vi "CheckGameBoardQueueLogic.vi"(8 "error in (no error)":errorcluster, 9 "Current Color in":i32, 10 "Coloring Board in":cluster{"tile":T1, "color":i8}[][](array[cluster]), 11 "Queue in":refnum<queue>) -> (0 "error out":errorcluster, 1 "Current Color out":i32, 2 "Coloring Board out":cluster{"tile":T1, "color":i8}[][](array[cluster]), 3 "Queue out":refnum<queue>)   [LabVIEW 2020]
uses:
  TypeDef/tiles-key-trunct.ctl
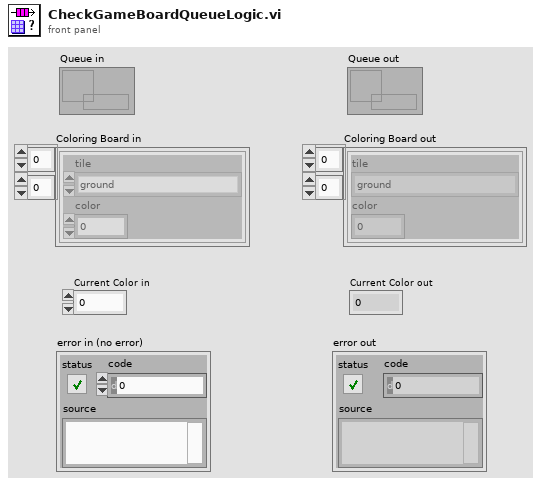
[diagram p1: front panel]
types:
  T1 = typedef "tiles-key-trunct.ctl" = enum16{"ground", "wall", "head (right)", "head (up)", "head (left)", "head (down)", "L-turn (right-up)", "L-turn (up-left)", "L-turn (left-down)", "L-turn (down-right)", "body (right)", "body (up)", "body (left)", "body (down)", "R-turn (right-down)", "R-turn (up-right)", "R-turn (left-up)", "R-turn (down-left)", "tail (right)", "tail (up)", "tail (left)", "tail (down)"}
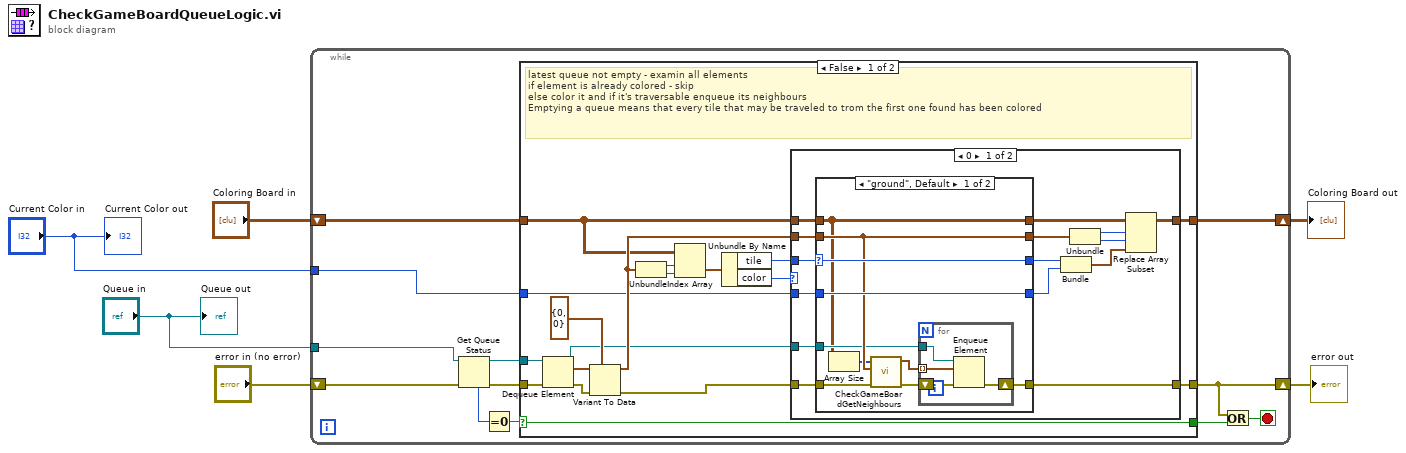
[diagram p0: block diagram]
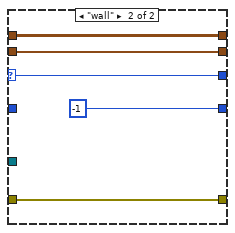
[diagram p2: hidden frame]
diagram:
  n1 = while {
    shift-right: [w11] -> w4
    shift-left: "error in (no error)" -> [w18]
    shift-right: [w14] -> w6
    shift-left: "Coloring Board in" -> [w13]
    tunnel: "Queue in" -> [w8]
    tunnel: "Current Color in" -> [w9]
    stop <- w10 stop-if-true
    n2 = Get Queue Status(queue=w8, error in (no error)=w18) -> (queue out=w7:refnum<queue>, error out=w15:errorcluster, # elements in queue=w17:i32)  [unwired: 1 in, 5 out]
    n3 = Equal To 0?(x=w17) -> (x = 0?=w16:bool)
    n4 = case shown="False" w16 {
      selector: w16 -> [w36 w73]
      tunnel: [w25 w75] -> w11
      tunnel: w15 -> [w34 w75]
      tunnel: [w19 w74] -> w14
      tunnel: w13 -> [w22 w74]
      tunnel: [w36 w73] -> w12
      tunnel: w7 -> [w35 _]
      tunnel: w9 -> [w20 _]
      frame False {
        # "latest queue not empty - examin all elements\nif element is already colored - skip \nelse color it and if it's traversable enqueue its neighbours\nEmptying a queue means that every tile that may be traveled to trom the first one found has been colored"
        n5 = Dequeue Element(queue=w35, error in (no error)=w34) -> (queue out=w21:refnum<queue>, element=w32:cluster{"row":i32, "col":i32}, error out=w33:errorcluster)  [unwired: 1 in, 1 out]
        n6 = Variant To Data(error in=w33, type=cluster{"row":i32, "col":i32} {"row"=0, "col"=0} ("cluster"), Variant=w32) -> (data=w23:cluster{"row":i32, "col":i32}, error out=w26:errorcluster)
        n7 = Unbundle(w23) -> ("row"=w30:i32, "col"=w29:i32)
        n8 = Index Array(array=w22, index (row)=w30, index (col)=w29) -> (element=w28:cluster{"tile":T1, "color":i8})
        n9 = Unbundle By Name(w28) -> ("tile"=w24:T1, "color"=w27:i8)
        n10 = case shown="0" w27 {
          tunnel: w26 -> [w51 w72]
          tunnel: [w50 w72] -> w25
          tunnel: w24 -> [w49 _]
          tunnel: w23 -> [w46 _]
          tunnel: w22 -> [w47 w71]
          tunnel: w21 -> [w48 _]
          tunnel: w20 -> [w45 _]
          tunnel: [w37 w71] -> w19
          frame 0 {
            n11 = case shown="\"ground\", Default" w49 {
              selector: w49 -> [w60 w66]
              tunnel: w51 -> [w59 w70]
              tunnel: [w55 w70] -> w50
              tunnel: w48 -> [w56 _]
              tunnel: [w52 w69] -> w44
              tunnel: w47 -> [w52 w69]
              tunnel: [w58 w68] -> w43
              tunnel: w46 -> [w58 w68]
              tunnel: w45 -> [w61 _]
              tunnel: [w61 -1] -> w39
              tunnel: [w60 w66] -> w40
              frame "ground", Default {
                n12 = Array Size(array=w52) -> (size(s)=w53:i32[])
                n13 = call "CheckGameBoardGetNeighbours.vi"("error in (no error)"=w59, "Position in"=w58, "Board size(s)"=w53) -> ("error out"=w57:errorcluster, "Positions out"=w54:cluster{"row":i32, "column":i32}[])  [unwired: 7 in]
                n14 = for {
                  tunnel: w54 -> [w63] mode=indexing
                  tunnel: w56 -> [w64]
                  shift-right: [w62] -> w55
                  shift-left: w57 -> [w65]
                  n15 = Enqueue Element(queue=w64, element=w63, error in (no error)=w65) -> (error out=w62:errorcluster)  [unwired: 1 in, 2 out]
                }
              }
              frame "wall" {
              }
            }
            n16 = Bundle("tile"=w40, "Current Color in"=w39) -> (w38:cluster{"tile":T1, "Current Color in":i32})  [unwired: 1 in]
            n17 = Unbundle(w43) -> ("row"=w42:i32, "col"=w41:i32)
            n18 = Replace Array Subset(array=w44, new element=w38, index (row)=w42, index (col)=w41) -> (w37:cluster{"tile":T1, "color":i8}[][])
          }
          frame 1, Default {
          }
        }
      }
      frame True {
        # "queue is empty - nothing to do here"
      }
    }
    n19 = Or(x=w11, y=w12) -> (x .or. y?=w10:bool)
  }
  "Coloring Board out" <- w6
  "error out" <- w4
  "Queue out" <- "Queue in"
  "Current Color out" <- "Current Color in"
